vi "VI Tree - numeric.vi"   [LabVIEW 2020]
uses:
  Random Number Within Range/Random Number Within Range - DBL.vi
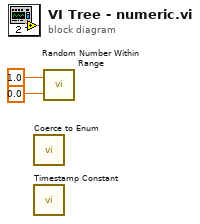
[diagram p0: block diagram]
diagram:
  n1 = call "Coerce to Enum.vi"() -> ()  [unwired: 1 in]
  n2 = call "Timestamp Constant.vi"() -> ()  [unwired: 1 in]
  n3 = call-poly "Random Number Within Range.vi"("High"=1.0 ("High (1.00)"), "Low"=0.0 ("Low (0.00)")) -> ()  [unwired: 3 in, 1 out]
